vi "随机数生成.vi"(9 "整数/浮点":bool, 10 "下限":dbl, 11 "上限":dbl) -> (3 "输出":dbl)   [LabVIEW 2012]
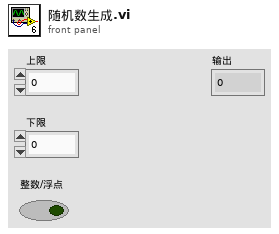
[diagram p1: front panel]
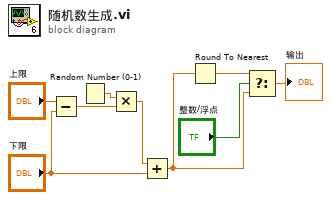
[diagram p0: block diagram]
diagram:
  n1 = Subtract(x="上限", y="下限") -> (x-y=w7:dbl)
  n2 = Random Number (0-1)() -> (number: 0 to 1=w9:dbl)
  n3 = Multiply(x=w9, y=w7) -> (x*y=w6:dbl)
  n4 = Add(x=w6, y="下限") -> (x+y=w2:dbl)
  n5 = Round To Nearest(number=w2) -> (nearest integer value=w3:dbl)
  n6 = Select(t=w3, s="整数/浮点", f=w2) -> (s? t:f=→"输出":dbl)
